vi "2 Waypoint Monitor.vi"() -> ()   [LabVIEW 2011]
doc: "Waypoint Monitor takes two things from the global variable - the list of waypoints and\nthe position of the robot at the time.\n\nIt compares the current position to the position of the current waypoint, and if that distance\nis less than the required accuracy the current waypoint value is incremented"
uses:
  0x2-OCU-Think Comm/0x2 Typedefs/Current Waypoint.ctl
  2 Classes/Waypoint/Waypoint.lvclass
  2 Globals/2 Global.vi
  2 Globals/2 Message Logger.vi
  2 Classes/MissionQueue/MissionQueue.lvclass
  2 Classes/Logger/Logger.lvclass
panel:
  out "Waypoint Tolerance":dbl
  out "Distance to waypoint":dbl
  # "Waypoint Monitor takes two things from the global variable - the list of waypoints and\nthe position of the robot at the time.\n\nIt compares the current position to the position of the current waypoint, and if that distance\nis less than the required accuracy the current waypoint value is incremented"
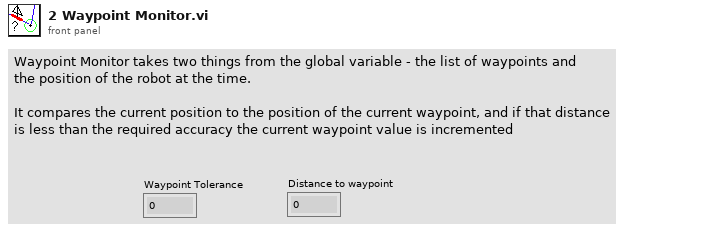
[diagram p1: front panel]
types:
  T1 = typedef "Current Waypoint.ctl" = i32
  T2 = typedef "Waypoints List.ctl" = refnum<class "Waypoint.lvclass">[]
  T3 = typedef "UTM Location.ctl" = cluster{"UTM Zone":dbl, "Hemisphere":enum16{"North", "South"}, "East":dbl, "North":dbl}
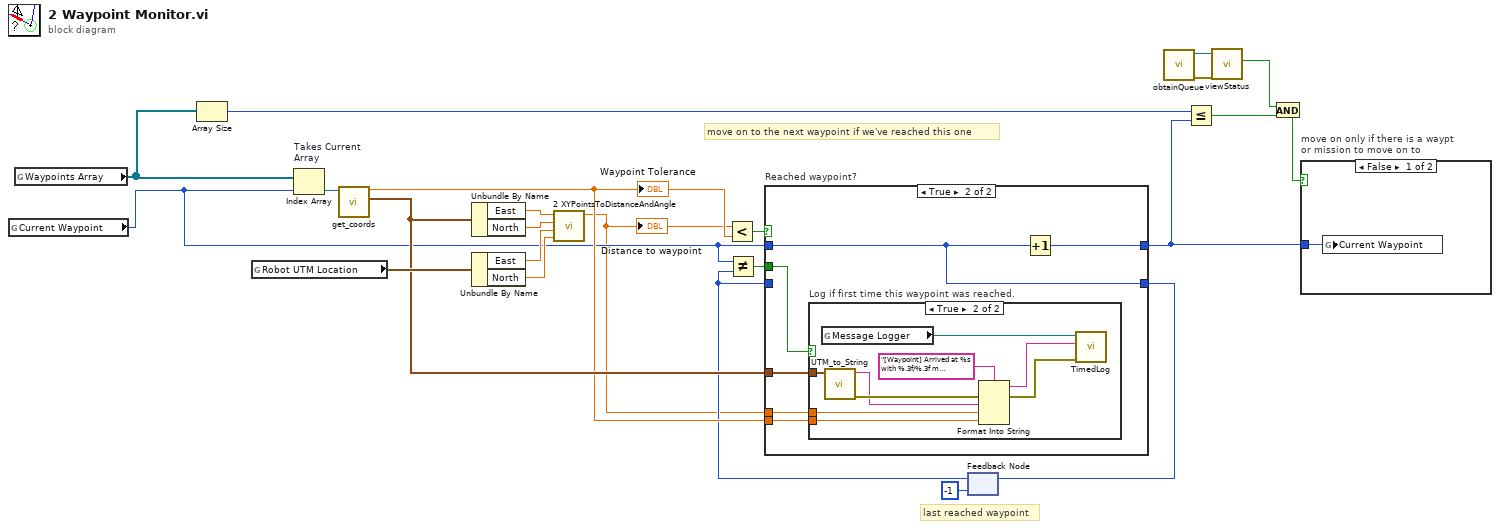
[diagram p0: block diagram]
diagram:
  # "last reached waypoint"
  # "move on to the next waypoint if we've reached this one"
  n1 = global read "2 Global.vi" "Current Waypoint"() -> (w4:T1)
  n2 = global read "2 Global.vi" "Waypoints Array"() -> (w23:T2)
  n3 = Array Size(array=w23) -> (size(s)=w15:i32)
  n4 = global read "2 Global.vi" "Robot UTM Location"() -> (w22:T3)
  n5 = Index Array "Takes Current\nArray"(array=w23, index=w4) -> (element=w17:refnum<class "Waypoint.lvclass">)
  n6 = call-dynamic "get_coords.vi"("Waypoint in"=w17) -> ("Tolerance (meters?)"=w7:dbl, "Coords"=w8:T3)  [unwired: 7 in, 2 out]
  "Waypoint Tolerance" <- w7
  n7 = Unbundle By Name(w8) -> ("East"=w19:dbl, "North"=w18:dbl)
  n8 = Unbundle By Name(w22) -> ("East"=w21:dbl, "North"=w20:dbl)
  n9 = call "2 XYPointsToDistanceAndAngle.vi"("East 2"=w20, "North 2"=w21, "East 1"=w18, "North 1"=w19) -> ("Distance"=w1:dbl)  [unwired: 6 in, 1 out]
  "Distance to waypoint" <- w1
  n10 = Less?(x=w1, y=w7) -> (x < y?=w16:bool)
  n11 = feedback #1(T1 -1 ("Current Waypoint")) -> (w3:T1)
  n12 = Not Equal?(x=w4, y=w3) -> (x != y?=w2:bool)
  n13 = case "Reached waypoint?" shown="True" w16 {
    tunnel: w4 -> [w25 w27]
    tunnel: [w25 w31] -> w14
    tunnel: w8 -> [_ w30]
    tunnel: w7 -> [_ w29]
    tunnel: w1 -> [_ w28]
    tunnel: [w24 w27] -> w6
    tunnel: w3 -> [w24 _]
    tunnel: w2 -> [_ w26]
    frame False {
    }
    frame True {
      n14 = case "Log if first time this waypoint was reached." shown="True" w26 {
        tunnel: w30 -> [_ w34]
        tunnel: w29 -> [_ w33]
        tunnel: w28 -> [_ w32]
        frame False {
        }
        frame True {
          n15 = global read "2 Message Logger.vi" "Message Logger"() -> (w40:refnum<class "Logger.lvclass">)
          n16 = call "UTM_to_String.vi"("UTM Location"=w34) -> ("error out"=w37:errorcluster, "UTM String"=w35:string)  [unwired: 9 in]
          n17 = Format Into String(format string="[Waypoint] Arrived at %s with %.3f/%.3f m tolerance.", error in=w37, w35, w32, w33) -> (resulting string=w38:string, error out=w39:errorcluster)  [unwired: 1 in]
          n18 = call "TimedLog.vi"("error in (no error)"=w39, "Message"=w38, "Logger in"=w40) -> ()  [unwired: 6 in, 3 out]
        }
      }
      n19 = Increment(x=w27) -> (x+1=w31:T1)
    }
  }
  n20 = feedback-in #1(w6) -> ()
  n21 = call "obtainQueue.vi"() -> ("Error Out"=w13:errorcluster, "MissionQueue.lvclass"=w9:refnum<class "MissionQueue.lvclass">)  [unwired: 10 in]
  n22 = Less Or Equal?(x=w15, y=w14) -> (x <= y?=w12:bool)
  n23 = call "viewStatus.vi"("error in (no error)"=w13, "MissionQueue in"=w9) -> ("Is empty?"=w10:bool)  [unwired: 6 in, 3 out]
  n24 = And(x=w10, y=w12) -> (x .and. y?=w11:bool)
  n25 = case "move on only if there is a waypt\nor mission to move on to" shown="False" w11 {
    tunnel: w14 -> [w41 _]
    frame False {
      n26 = global write "2 Global.vi" "Current Waypoint"(w41) -> ()
    }
    frame True {
    }
  }
